vi "LS330_Read_Range.vi"(8 "error in":errorcluster, 10 "Heater":string(combo)="1", 11 "VISA resource name":refnum<visa-resource-name>) -> (0 "error out":errorcluster, 2 "Range":T1, 3 "VISA resource name out":refnum<visa-resource-name>)   [LabVIEW 2021]
uses:
  Heater_Range.ctl
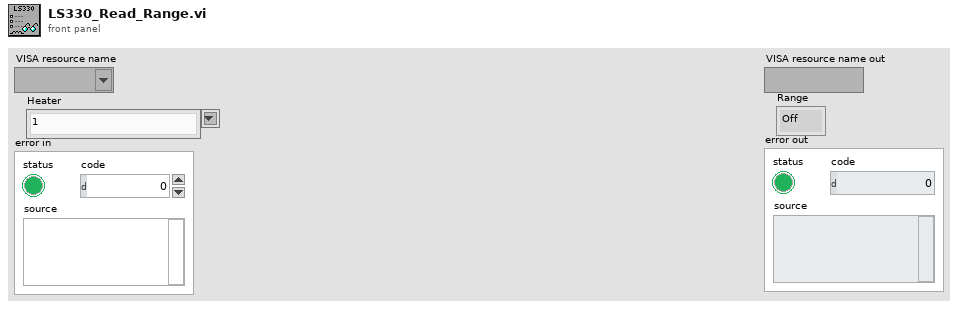
[diagram p1: front panel]
types:
  T1 = typedef "Heater_Range.ctl" = enum16{"Off", "Low", "Medium", "High"}
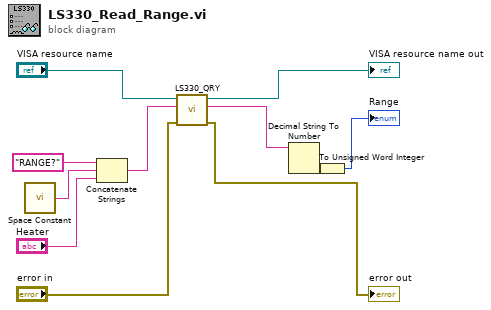
[diagram p0: block diagram]
diagram:
  n1 = call <vilib>:"Space Constant.vi"() -> ("String"=w9:string)
  n2 = Concatenate Strings("RANGE?" ("string"), w9, "Heater") -> (w7:string)
  n3 = call "LS330_QRY.vi"("error in"="error in", "CMD"=w7, "VISA resource name"="VISA resource name") -> ("error out"=→"error out":errorcluster, "OUT"=w4:string, "VISA resource name out"=→"VISA resource name out":refnum<visa-resource-name>)  [unwired: 5 in, 1 out]
  n4 = Decimal String To Number(string=w4) -> (number=w2:i32)  [unwired: 2 in, 1 out]
  n5 = To Unsigned Word Integer(number=w2) -> (unsigned 16bit integer=→"Range":u16)
